vi "NewPanelCompare.vi"(10 "TipPanel":refnum<class "TipPanel.lvclass">, 11 "loop data in":T1) -> (1 "Same exact Panel?":bool, 2 "Same Panel Type?":bool, 3 "loop data out":T1)   [LabVIEW 2021, in "TipStripOOPanel.lvlib"]
uses:
  TipStripOOPanel.lvlib
  Loop Data Parent.ctl
  Classes/TipPanel/TipPanel.lvclass
  <vilib>/IlluminatedG/IG OOPanel/OOPanel/Manager/Manager.lvclass
  PanelMap.ctl
  PanelMapData.ctl
  Classes/TipPanel/ToPanelUEWrapper.ctl
  Classes/TipPanel/ToPanelUE.ctl
  <vilib>/Futures/Futures/Promise/Promise.lvclass
  refs.ctl
  content size.ctl
  <vilib>/Utility/miscctls.llb/LVRectTypeDef.ctl
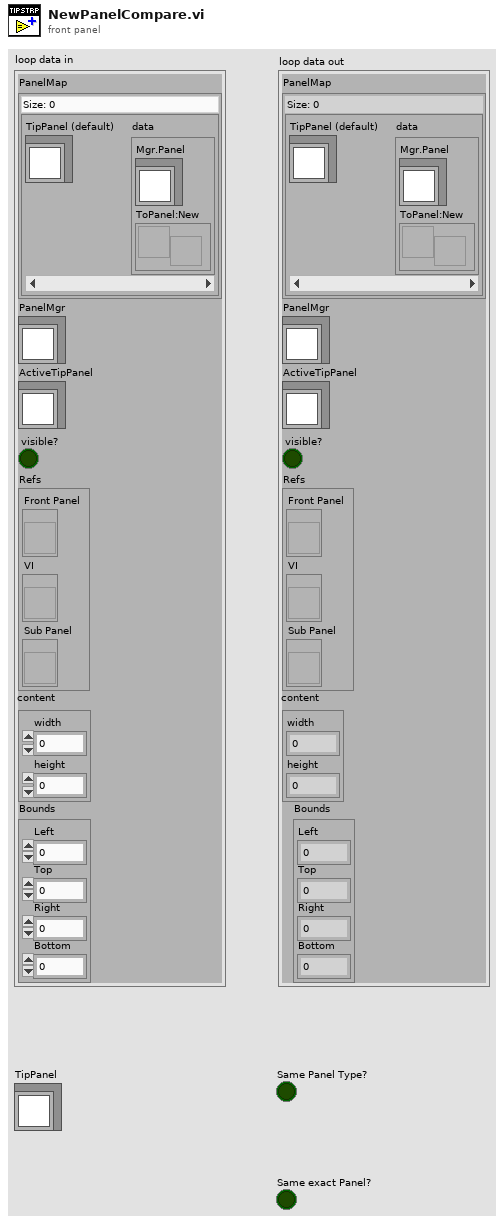
[diagram p1: front panel]
types:
  T1 = typedef "TipStripOOPanel.lvlib/Loop Data Parent.ctl" = cluster{"PanelMap":T2, "PanelMgr":refnum<class "Manager.lvclass">, "ActiveTipPanel":refnum<class "TipPanel.lvclass">, "visible?":bool, "Refs":T4, "content":T5, "Bounds":T6}
  T2 = typedef "TipStripOOPanel.lvlib/PanelMap.ctl" = map{refnum<class "TipPanel.lvclass">, T3}
  T3 = typedef "TipStripOOPanel.lvlib/PanelMapData.ctl" = cluster{"Mgr.Panel":refnum<class "TipPanel.lvclass">, "ToPanel:New":refnum<user-event>}
  T4 = typedef "TipStripOOPanel.lvlib/refs.ctl" = cluster{"Front Panel":refnum<vi>, "VI":refnum<vi>, "Sub Panel":refnum<vi>}
  T5 = typedef "TipStripOOPanel.lvlib/content size.ctl" = cluster{"width":i32, "height":i32}
  T6 = typedef "LVRectTypeDef.ctl" = cluster{"Left":i16, "Top":i16, "Right":i16, "Bottom":i16}
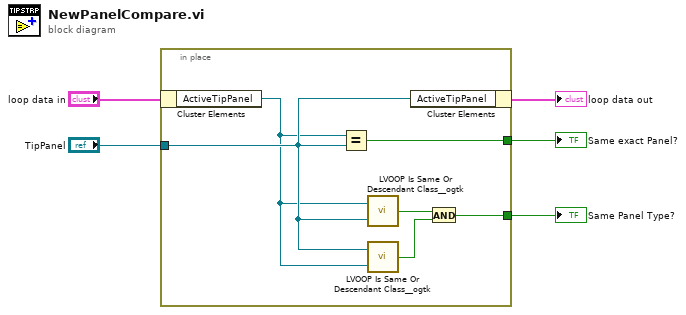
[diagram p0: block diagram]
diagram:
  n1 = in-place {
    in-place-border: "TipPanel" -> [w10]
    in-place-border: [w11] -> w2
    in-place-border: [w6] -> w1
    n2 = in-place-cluster #1("loop data in") -> ("ActiveTipPanel"=w9:refnum<class "TipPanel.lvclass">)
    n3 = Equal?(x=w9, y=w10) -> (x = y?=w11:bool)
    n4 = call <userlib>:"LVOOP Is Same Or Descendant Class__ogtk.vi"("Possible Descendant Object"=w10, "Object"=w9) -> ("Is Same Class or Descendant?"=w8:bool)
    n5 = call <userlib>:"LVOOP Is Same Or Descendant Class__ogtk.vi"("Possible Descendant Object"=w9, "Object"=w10) -> ("Is Same Class or Descendant?"=w7:bool)
    n6 = in-place-cluster #1("ActiveTipPanel"=w10) -> (→"loop data out":T1)
    n7 = And(x=w8, y=w7) -> (x .and. y?=w6:bool)
  }
  "Same exact Panel?" <- w2
  "Same Panel Type?" <- w1
